vi "ESR Scanner - pulsed optimizer - stop-able.vi"(0 "ESR Parameters":T1={"Window 1 time (s)"=0.012, "Window 2 time (s)"=5e-06, "Window 3 time (s) "=0.02, "Window 4 time (s)"=5e-07, "Window 4 channels"=[TRUE, FALSE, FALSE, TRUE], "Window 3 channels"=[TRUE, FALSE, TRUE, TRUE], "Window 2 channels"=[TRUE, FALSE, FALSE, TRUE], "Window 1 channels"=[TRUE, TRUE, FALSE, TRUE], "Path to ESR Burner"=path "C:/Users/Loncar/Desktop/ESR VIs - Srujan/Sam Kim/PB/ESRFreq.exe"}, 1 "MW start freq (GHz)":dbl=2.84, 2 "MW stop freq (GHz)":dbl=2.9, 3 "# freq points":i32=61, 4 "# scans before track":i32=50, 5 "#scan iterations":i32=50, 6 "IntGraph Refnum":refnum<vi>, 7 "Optimize Parameters":T2={"Volt Step"={"X"=0.01, "Y"=0.01, "Z"=0.0}, "Num Iterations"=1, "Dwell Time (ms)"=100, "Volts Range"={"X"=0.1, "Y"=0.1, "Z"=0.0}} {"Volts Range"."Z" min=0.0; "Volts Range"."Y" min=0.0; "Volts Range"."X" min=0.0; "Dwell Time (ms)" min=0; "Num Iterations" min=1 step=1; "Volt Step"."Z" min=0.0; "Volt Step"."Y" min=1e-06; "Volt Step"."X" min=1e-06}, 8 "XY Graph Refnum":refnum<vi>, 14 "Save avg spectrum data to spreadsheet?":bool, 15 "Path for avg spectrum spreadsheet":path=path "C:/experiment/data/may_15_2012/SIL1_NV1_pippin_uW_off", 16 "Save avg spectrum graph?":bool, 17 "Path for avg spectrum graph":path=path "C:/experiment/data/may_15_2012/SIL1_NV1_pippin_uW_off") -> ()   [LabVIEW 2012]
uses:
  <vilib>/Analysis/NI_AALBase.lvlib
  <vilib>/Analysis/baseanly.llb/Mean (DBL).vi
  <vilib>/Utility/file.llb/Write To Spreadsheet File (DBL).vi
  <vilib>/DAQmx/read.llb/DAQmx Read (Counter 1D U32 1Chan NSamp).vi
  Channels.vi
  Global Vars.vi
  Strict Type Def - Optimize Parameters Cluster.ctl
  ESR Window Parameters.ctl
panel:
  in  "stop":bool
  out "Counts vs. frequency":i32[][](graph)
  out "Avg ESR spectrum":cluster{"Y":dbl[], "Y":dbl[]}[](graph)
  # "Note:\nThis is not a standalone program. It is called from ScannerUI"
  # "Default PB connections:\nPB0 - MW switch\nPB1 - MW freq step\nPB2 - Counter sample clk\nPB3 - Green AOM"
  # "VI for ESR spectrum measurement\n08/26/2013, Srujan Meesala"
  # "Stop experiment and\nreset PulseBlaster"
  # "MW freq step\ndwell time"
  # "MW freq step"
  # "Wait"
  # "Fluorescence\ncounting"
  # "Ctr sample clk"
  # "Wait"
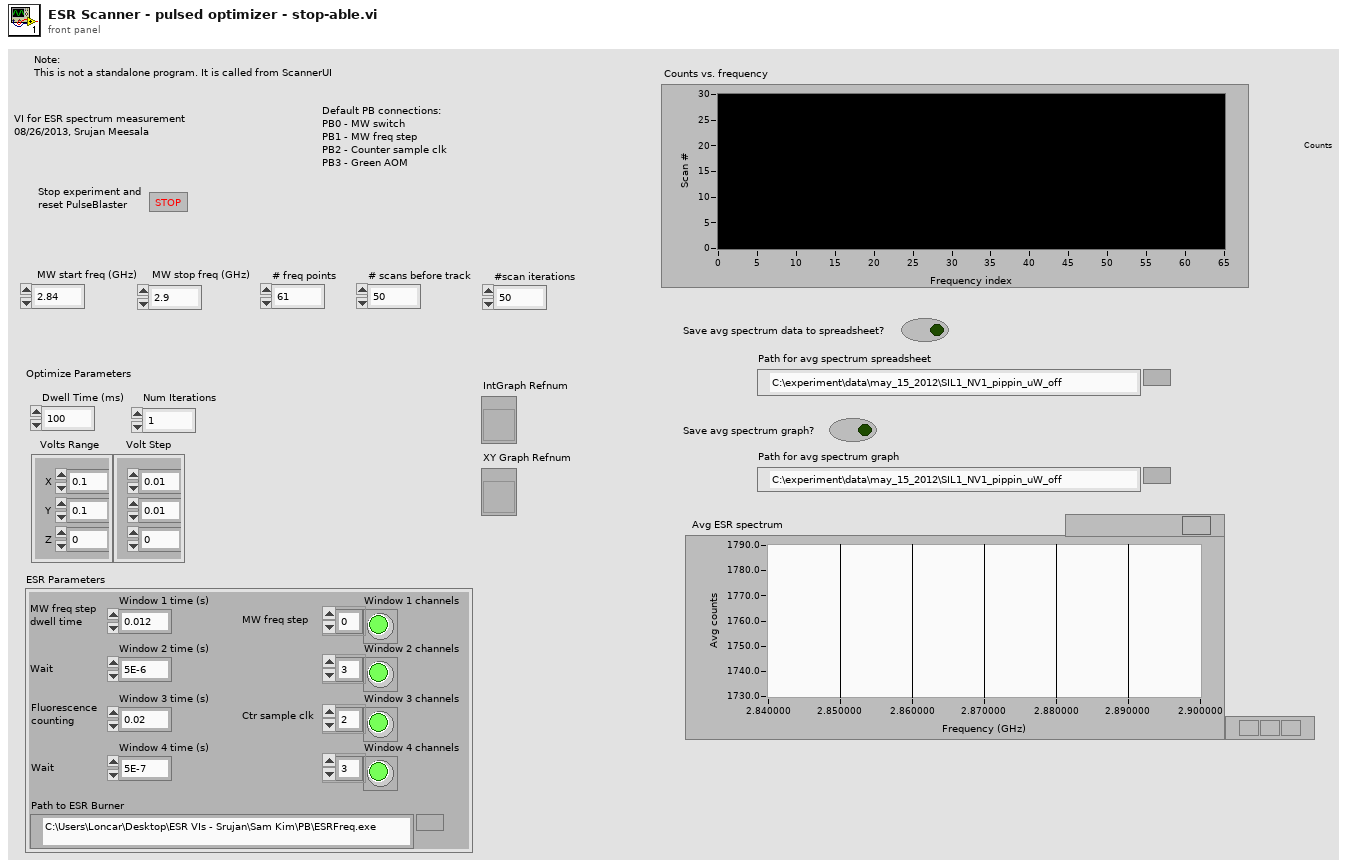
[diagram p1: front panel]
types:
  T1 = typedef "ESR Window Parameters.ctl" = cluster{"Window 1 time (s)":dbl, "Window 2 time (s)":dbl, "Window 3 time (s) ":dbl, "Window 4 time (s)":dbl, "Window 4 channels":bool[], "Window 3 channels":bool[], "Window 2 channels":bool[], "Window 1 channels":bool[], "Path to ESR Burner":path}
  T2 = typedef "Strict Type Def - Optimize Parameters Cluster.ctl" = cluster{"Volt Step":cluster{"X":dbl, "Y":dbl, "Z":dbl}, "Num Iterations":i32, "Dwell Time (ms)":i32, "Volts Range":cluster{"X":dbl, "Y":dbl, "Z":dbl}}
  T3 = typedef "imagedata.ctl" = cluster{"image type":i32, "image depth":i32, "image":u8[], "mask":u8[], "colors":u32[], "Rectangle":cluster{"left":i16, "top":i16, "right":i16, "bottom":i16}}
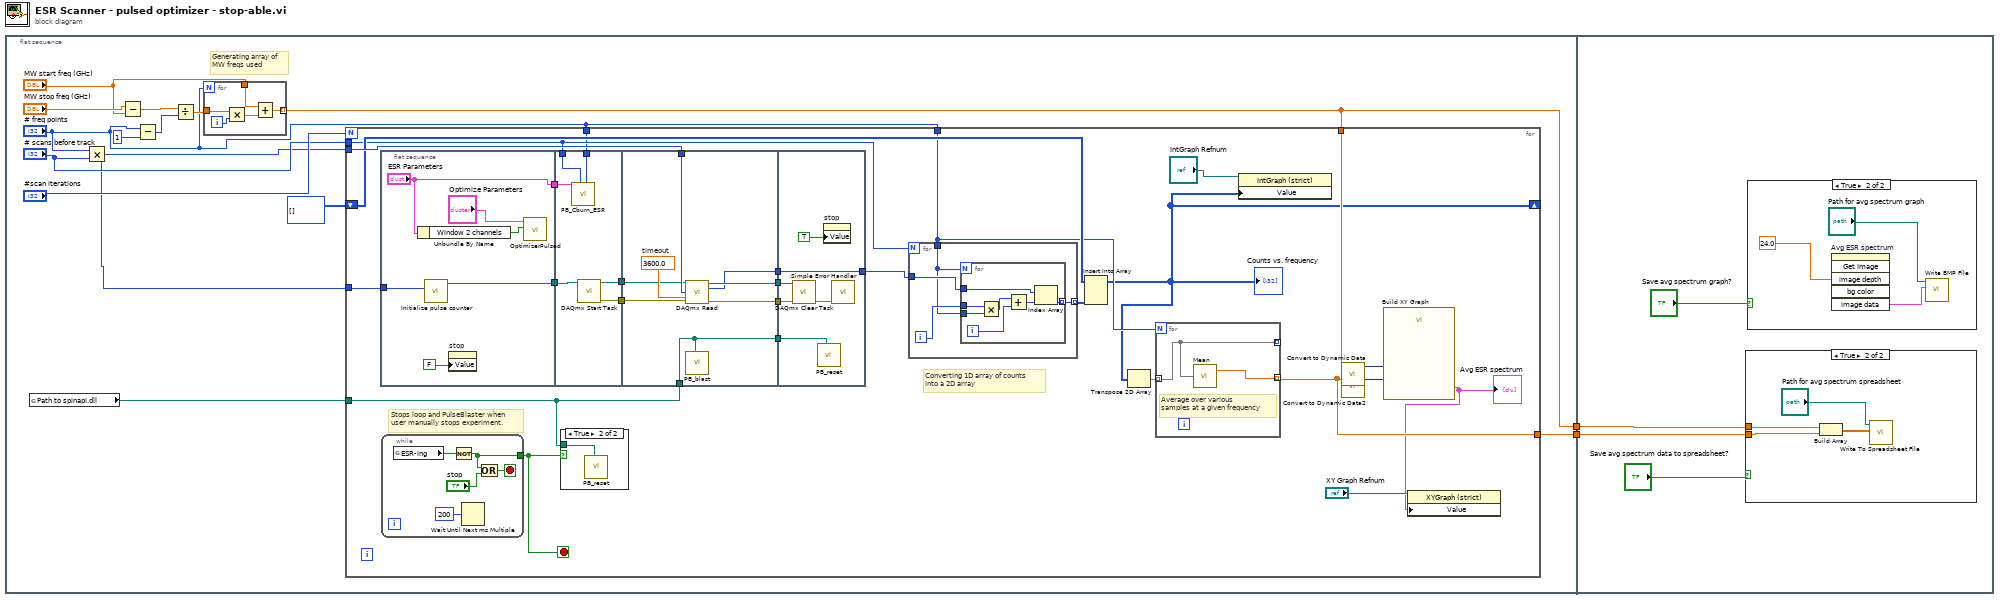
[diagram p0: block diagram]
diagram:
  n1 = flat-sequence {
    tunnel: [w8] -> w2
    tunnel: [w7] -> w1
    tunnel: w2 -> [w96]
    tunnel: w1 -> [w95]
    frame #0 {
      # "Generating array of\nMW freqs used"
      n2 = global read "Channels.vi" "Path to spinapi.dll"() -> (w5:path)
      n3 = Multiply(x="# freq points", y="# scans before track") -> (x*y=w3:i32)
      n4 = Subtract(x="MW stop freq (GHz)", y="MW start freq (GHz)") -> (x-y=w14:dbl)
      n5 = Subtract(x="# freq points", y=u32 1 ("Reset Count")) -> (x-y=w15:u32)
      n6 = Divide(x=w14, y=w15) -> (x/y=w12:dbl)
      n7 = for {
        N: "# freq points" -> [_]
        tunnel: w12 -> [w93]
        tunnel: "MW start freq (GHz)" -> [w91]
        tunnel: [w90] -> w8 mode=indexing
        i -> [w94]
        n8 = Multiply(x=w93, y=w94) -> (x*y=w92:dbl)
        n9 = Add(x=w91, y=w92) -> (x+y=w90:dbl)
      }
      n10 = for {
        N: "#scan iterations" -> [_]
        tunnel: w5 -> [w25]
        tunnel: w3 -> [w44]
        tunnel: "# scans before track" -> [w23]
        tunnel: "# freq points" -> [w32]
        shift-right: [w28] -> _
        shift-left: i32[][] [] ("Flourescence Data") -> [w34]
        tunnel: w8 -> [w31]
        tunnel: [w30] -> w7
        tunnel: "# freq points" -> [w22]
        tunnel: w3 -> [w19]
        stop <- w17 stop-if-true
        # "Stops loop and PulseBlaster when\nuser manually stops experiment."
        # "Converting 1D array of counts \ninto a 2D array"
        n11 = flat-sequence {
          tunnel: ["ESR Parameters"] -> w24
          tunnel: w19 -> [w68]
          tunnel: [w67] -> w18
          tunnel: w24 -> [w71]
          tunnel: w23 -> [w73]
          tunnel: w22 -> [w72]
          tunnel: [w75] -> w21
          tunnel: [w74] -> w20
          tunnel: w18 -> [w70]
          tunnel: w44 -> [w82]
          tunnel: w25 -> [w79]
          tunnel: [w81] -> w43
          tunnel: [w80] -> w42
          tunnel: [w79] -> w41
          tunnel: [w78] -> w37
          tunnel: [w78] -> w36
          tunnel: w21 -> [w77]
          tunnel: w20 -> [w76]
          tunnel: w43 -> [w86]
          tunnel: w42 -> [w87]
          tunnel: w41 -> [w89]
          tunnel: [w88] -> w35
          tunnel: w37 -> [w88]
          tunnel: w36 -> [_]
          frame #0 {
            n12 = Unbundle By Name("ESR Parameters") -> ("Window 2 channels"=w66:bool[])
            n13 = call "Initialize pulse counter.vi"("Samples per channel"=w68) -> ("DAQmx Task Name"=w67:refnum<k21>)  [unwired: 9 in, 1 out]
            n14 = property on="stop" class="Bool (strict)"("Value"=FALSE) -> ()  [unwired: 2 in, 2 out]
            n15 = call "OptimizerPulsed.vi"("Optimize active channels"=w66, "Optimize Parameters"="Optimize Parameters") -> ()  [unwired: 9 in, 1 out]
          }
          frame #1 {
            n16 = call "PB_Cburn_ESR.vi"("# freq points"=w72, "# scans before track"=w73, "ESR Parameters"=w71) -> ()  [unwired: 9 in]
            n17 = call <vilib>:"DAQmx Start Task.vi"("task/channels in"=w70) -> ("task out"=w75:refnum<k21>, "error out"=w74:errorcluster)  [unwired: 13 in]
          }
          frame #2 {
            w83 = 3600.0  # timeout
            n18 = call-poly <vilib>:"DAQmx Read.vi"("task/channels in"=w77, "number of samples per channel"=w82, "timeout"=w83, "error in"=w76) -> ("task out"=w80:refnum<k21>, "data"=w78:u32[], "error out"=w81:errorcluster)  [unwired: 9 in]
            n19 = call "PB_blast.vi"("Path to spinapi.dll"=w79) -> ()  [unwired: 7 in]
          }
          frame #3 {
            n20 = call <vilib>:"DAQmx Clear Task.vi"("task in"=w87, "error in"=w86) -> ("error out"=w85:errorcluster)  [unwired: 13 in]
            n21 = call "PB_reset.vi"("Path to spinapi.dll"=w89) -> ()  [unwired: 7 in]
            n22 = property on="stop" class="Bool (strict)"("Value"=TRUE) -> ()  [unwired: 2 in, 2 out]
            n23 = call <vilib>:"Simple Error Handler.vi"("error in (no error)"=w85) -> ()  [unwired: 4 in, 5 out]
          }
        }
        n24 = while {
          tunnel: [w46] -> w17
          stop <- w47 stop-if-true
          n25 = global read "Global Vars.vi" "ESR-ing"() -> (w49:bool)
          n26 = Not(x=w49) -> (.not. x?=w46:bool)
          n27 = Wait Until Next ms Multiple(millisecond multiple=u32 200) -> ()  [unwired: 1 out]
          n28 = Or(x=w46, y="stop") -> (x .or. y?=w47:bool)
        }
        n29 = case shown="True" w17 {
          tunnel: w25 -> [_ w50]
          frame False {
          }
          frame True {
            n30 = call "PB_reset.vi"("Path to spinapi.dll"=w50) -> ()  [unwired: 7 in]
          }
        }
        n31 = for {
          N: w23 -> [_]
          tunnel: w35 -> [w54]
          tunnel: w32 -> [w51]
          tunnel: [w53] -> w33 mode=indexing
          i -> [w52]
          n32 = for {
            N: w51 -> [_]
            tunnel: w52 -> [w61]
            tunnel: w54 -> [w59]
            tunnel: [w58] -> w53 mode=indexing
            tunnel: w51 -> [w56]
            i -> [w57]
            n33 = Multiply(x=w61, y=w56) -> (x*y=w55:i32)
            n34 = Add(x=w55, y=w57) -> (x+y=w60:i32)
            n35 = Index Array(array=w59, index=w60) -> (element=w58:u32)
          }
        }
        n36 = Insert Into Array(array=w34, new element=w33) -> (w28:i32[][])  [unwired: 2 in]
        "Counts vs. frequency" <- w28
        n37 = Transpose 2D Array(2D array=w28) -> (transposed array=w38:i32[][])
        n38 = for {
          N: w32 -> [_]
          tunnel: [w62] -> _ mode=indexing
          tunnel: [w63] -> w30 mode=indexing
          tunnel: w38 -> [w62] mode=indexing
          # "Average over various \nsamples at a given frequency"
          n39 = call-poly <vilib>:"Mean.vi"("X"=w62) -> ("mean"=w63:dbl)  [unwired: 1 out]
        }
        n40 = property class="IntGraph (strict)"(reference="IntGraph Refnum", "Value"=w28) -> ()  [unwired: 1 in, 2 out]
        n41 = call "Convert to Dynamic Data"("Array"=w31) -> ("Dynamic Data Type"=w40:dynamicdata)  [unwired: 3 in]
        n42 = call "Convert to Dynamic Data2"("Array"=w30) -> ("Dynamic Data Type"=w39:dynamicdata)  [unwired: 3 in]
        n43 = call "Build XY Graph"("Y Input"=w39, "X Input"=w40) -> ("XY Graph"=w26:cluster{"Y":dbl[], "Y":dbl[]}[])  [unwired: 3 in, 6 out]
        "Avg ESR spectrum" <- w26
        n44 = property class="XYGraph (strict)"(reference="XY Graph Refnum", "Value"=w26) -> ()  [unwired: 1 in, 2 out]
      }
    }
    frame #1 {
      n45 = case shown="True" "Save avg spectrum data to spreadsheet?" {
        tunnel: w96 -> [_ w100]
        tunnel: w95 -> [_ w99]
        frame False {
        }
        frame True {
          n46 = Build Array(w100, w99) -> (w101:dbl[][])
          n47 = call-poly <vilib>:"Write To Spreadsheet File.vi"("2D data"=w101, "file path (dialog if empty)"="Path for avg spectrum spreadsheet") -> ()  [unwired: 6 in, 1 out]
        }
      }
      n48 = case shown="True" "Save avg spectrum graph?" {
        frame False {
        }
        frame True {
          n49 = invoke on="Avg ESR spectrum" class="XYGraph (strict)" method="Get Image"("image depth"=24.0 ("Initial Delay")) -> ("image data"=w103:T3)  [unwired: 5 in, 5 out]
          n50 = call <vilib>:"Write BMP File.vi"("image data"=w103, "path to BMP file"="Path for avg spectrum graph") -> ()  [unwired: 8 in, 2 out]
        }
      }
    }
  }
